vi "Error Query.vi"() -> ()   [LabVIEW 2020, in "CTI-Scratchpad.lvlib"]
uses:
  CTI-Scratchpad.lvlib
  CTI/Session/Session.lvclass
  CTI/VisaComms/VisaComms.lvclass
panel:
  out "error out":errorcluster
  in  "Port":refnum<visa-resource-name>="COM3"
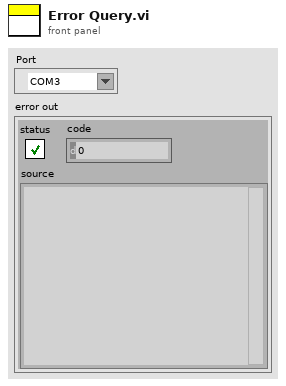
[diagram p1: front panel]
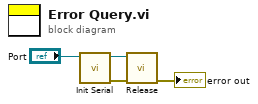
[diagram p0: block diagram]
diagram:
  n1 = call "Init Serial.vi"("VISA resource name in"="Port") -> ("error out"=w1:errorcluster, "Session"=w2:refnum<class "Session.lvclass">)  [unwired: 8 in, 1 out]
  n2 = call-dynamic "Release.vi"("error in (no error)"=w1, "Session in"=w2) -> ("error out"=→"error out":errorcluster)  [unwired: 9 in]
